vi "Stop Core.vi"(10 "final error code":i32, 11 "Elevator Controller Actor in":refnum<class "Sim Display Console Actor.lvclass">) -> (3 "Elevator Controller Actor out":refnum<class "Sim Display Console Actor.lvclass">)   [LabVIEW 2022 SP3, in "Sim Display Console Actor.lvlib" / "Sim Display Console Actor.lvclass"]
doc: "(<B>Filename</B>: Actor Framework.lvlib:Actor.lvclass:Stop Core.vi)\n\nDefines what the actor does before it stops. Use the <B>final error code</B> input to determine whether the actor shut down in response to an error.\n\nBy default, this method does nothing. A descendant class may override it to define behavior, such as shutting down any processes the actor initiated in its override of the Actor Core method."
uses:
  Sim Display Console Actor.lvclass
  Sim Display Console Actor.lvclass/Sim Display Console Actor.ctl
  Display Console Actor/Display Console Actor/Display Console Actor.lvclass
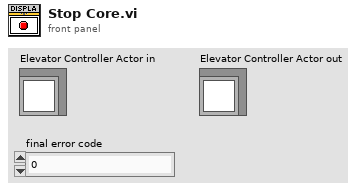
[diagram p1: front panel]
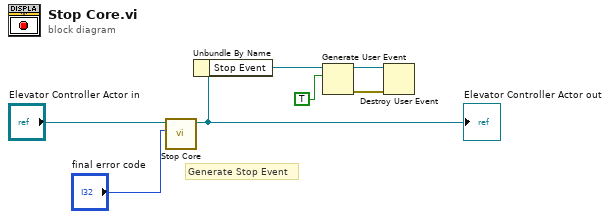
[diagram p0: block diagram]
diagram:
  # "Generate Stop Event"
  n1 = call-parent "Stop Core.vi"("final error code"="final error code", "Actor in"="Elevator Controller Actor in") -> ("Actor out"=w3:refnum<class "Sim Display Console Actor.lvclass">)  [unwired: 9 in]
  "Elevator Controller Actor out" <- w3
  n2 = Unbundle By Name(w3) -> ("Stop Event"=w2:refnum<user-event>)
  n3 = Generate User Event(user event=w2, event data cluster=TRUE ("event data")) -> (user event out=w5:refnum<user-event>, error out=w4:errorcluster)  [unwired: 2 in]
  n4 = Destroy User Event(user event=w5, error in=w4) -> ()  [unwired: 1 out]
